vi "SFCS_ChkRout.vi"(5 "URL":string) -> (1 "Status":string)   [LabVIEW 2011]
uses:
  Instance           4 29Saved   SFCS_ChkRoute_ComCode .vi
  Instance           1 29Saved   SFCS_ChkRoute_ComCode .vi
  Instance           2 29Saved   SFCS_ChkRoute_ComCode .vi
  Instance           3 29Saved   SFCS_ChkRoute_ComCode .vi
  data/MCSDLL.dll
panel:
  out "軟體版本Software Version":string
  out "Begin time":u32
  out "SFCS System Enable":string
  out "STAGE":string
  out "Unit SN":string
  out "USN_Length":i32
  out "SFCS_IP":string
  # "SFCS Check Route"
  # "2015-3-27"
  # "SFCS的網址"
  # "站名"
  # "序號"
  # "訊息"
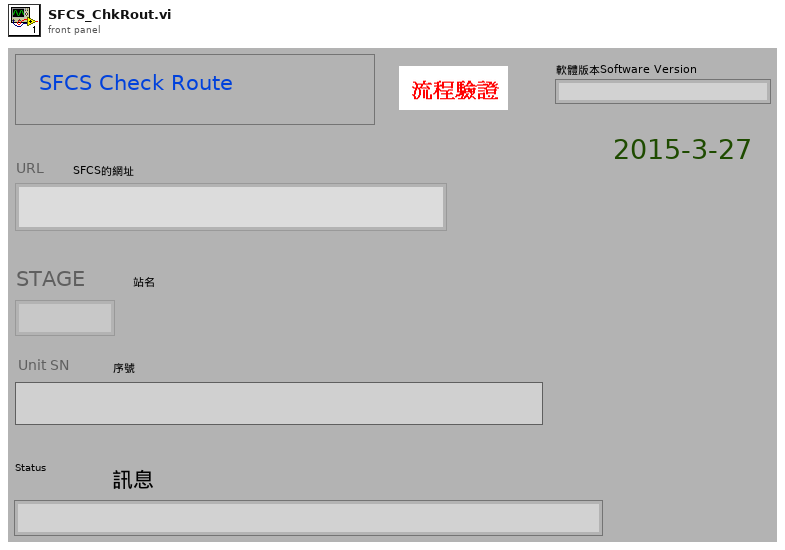
[diagram p1: front panel]
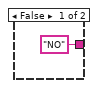
[diagram p5: hidden frame]
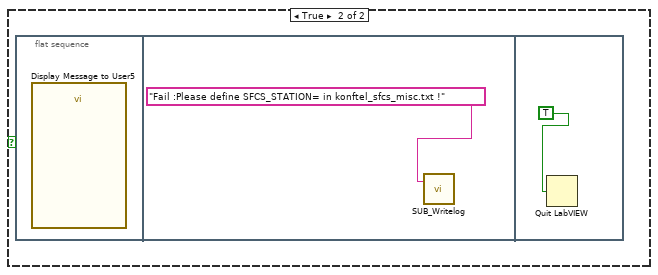
[diagram p8: hidden frame]
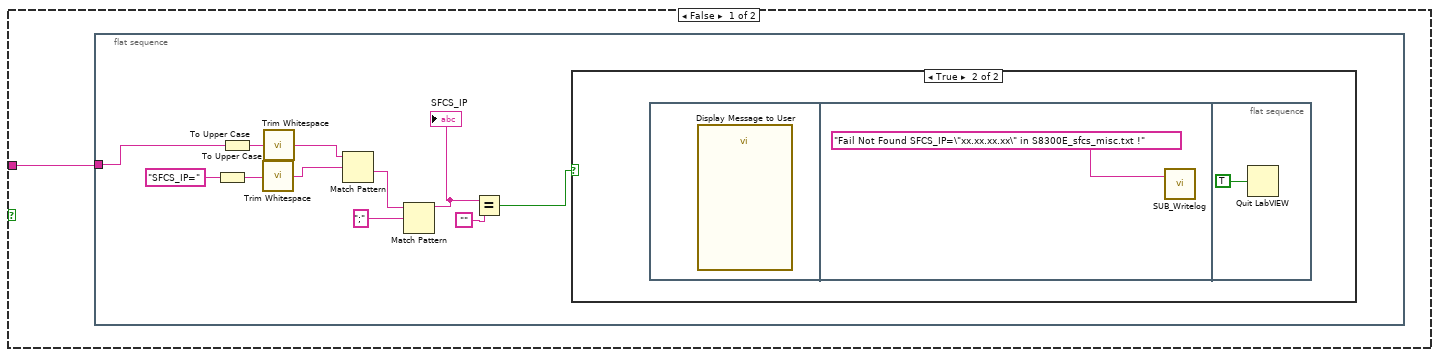
[diagram p10: hidden frame]
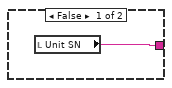
[diagram p12: hidden frame]
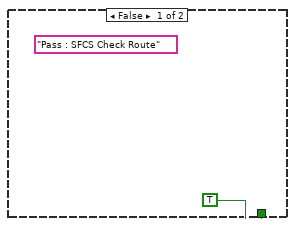
[diagram p13: hidden frame]
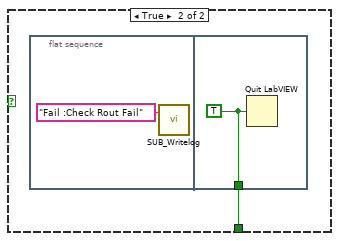
[diagram p14: hidden frame]
diagram:
  n1 = flat-sequence {
    frame #0 {
      n2 = Tick Count (ms)() -> (millisecond timer value=→"Begin time":u32)
    }
    frame #1 {
      n3 = call "SUB_SW_Version.vi"() -> ("Current Software Version"=→"軟體版本Software Version":string)  [unwired: 3 in]
      n4 = local write "Unit SN"("") -> ()
    }
    frame #2 {
      n5 = call "SUB_ReadScript_File.vi"("Script FileName"="barcode.log" ("name or relative path")) -> ("text"=w4:string, "error out"=w7:errorcluster)  [unwired: 1 in, 1 out]
      n6 = Unbundle(w7) -> ("code"=w6:i32)  [unwired: 2 out]
      n7 = Equal To 0?(x=w6) -> (x = 0?=w5:bool)
      n8 = case shown="True" w5 {
        tunnel: w4 -> [_ w11]
        frame False {
        }
        frame True {
          n9 = call "SUB_FindSpecificString.vi"("Find this String"="PRODUCT_SN=", "String data"=w11) -> ("before \"; \" string"=w9:string, "Found"=w10:bool)  [unwired: 2 in]
          n10 = case shown="True" w10 {
            tunnel: w9 -> [_ w13]
            frame False {
            }
            frame True {
              n11 = local write "Unit SN"(w13) -> ()
            }
          }
        }
      }
    }
    frame #3 {
      # "Check SFCS Enable in Mojo_script.txt"
      n12 = call "SUB_ReadScript_File.vi"("Script FileName"="S8300E_sfcs_misc.txt") -> ("text"=w19:string, "error out"=w16:errorcluster)  [unwired: 1 in, 1 out]
      n13 = Unbundle By Name(w16) -> ("code"=w17:i32)
      n14 = Equal To 0?(x=w17) -> (x = 0?=w18:bool)
      n15 = case shown="True" w18 {
        tunnel: w19 -> [_ w27]
        tunnel: ["NO" ("before \"; \" string") w25] -> w20
        frame False {
        }
        frame True {
          n16 = call "SUB_FindSpecificString.vi"("Find this String"="SFCS_SYSTEM_ENABLE=", "String data"=w27) -> ("before \"; \" string"=w25:string)  [unwired: 2 in, 1 out]
          "SFCS System Enable" <- w25
        }
      }
      n17 = Equal?(x=w20, y="YES") -> (x = y?=w15:bool)
      n18 = case shown="False" w15 {
        frame False {
          n19 = flat-sequence {
            frame #0 {
              n20 = call "SUB_Writelog.vi"("Pass/Fail"="Done :SFCS_ChkRoute_ComCode by PASS!") -> ()  [unwired: 2 in]
            }
            frame #1 {
              n21 = Quit LabVIEW(quit? (T)=TRUE) -> ()
            }
          }
        }
        frame True {
        }
      }
    }
    frame #4 {
      n22 = case shown="True" FALSE {
        frame False {
        }
        frame True {
          n23 = call "SUB_DELETE_SpecificFile.vi"("Filename to be  Deleted"="SFCS_INFO.LOG") -> ()  [unwired: 2 in, 1 out]
        }
      }
    }
    frame #5 {
      n24 = call "SUB_ReadScript_File.vi"("Script FileName"="S8300E_sfcs_misc.txt") -> ("text"=w31:string, "error out"=w34:errorcluster)  [unwired: 1 in, 1 out]
      n25 = Unbundle By Name(w34) -> ("code"=w33:i32)
      n26 = Equal To 0?(x=w33) -> (x = 0?=w32:bool)
      n27 = case shown="True" w32 {
        tunnel: w31 -> [_ w35]
        frame False {
        }
        frame True {
          n28 = To Upper Case(1:"SFCS_USNLength=" ("string")) -> (0:w44:string)
          n29 = To Upper Case(1:w35) -> (0:w46:string)
          n30 = call <vilib>:"Trim Whitespace.vi"("string"=w44) -> ("trimmed string"=w42:string)  [unwired: 1 in]
          n31 = call <vilib>:"Trim Whitespace.vi"("string"=w46) -> ("trimmed string"=w45:string)  [unwired: 1 in]
          n32 = Match Pattern(string=w45, regular expression=w42) -> (after substring=w40:string)  [unwired: 1 in, 3 out]
          n33 = Match Pattern(string=w40, regular expression=";") -> (before substring=w37:string)  [unwired: 1 in, 3 out]
          n34 = Equal?(x=w37, y="") -> (x = y?=w38:bool)
          n35 = Decimal String To Number(string=w37) -> (number=→"USN_Length":i32)  [unwired: 2 in, 1 out]
          n36 = case shown="False" w38 {
            tunnel: w35 -> [w50 _]
            frame False {
              n37 = To Upper Case(1:"SFCS_STATION=" ("string")) -> (0:w55:string)
              n38 = To Upper Case(1:w50) -> (0:w57:string)
              n39 = call <vilib>:"Trim Whitespace.vi"("string"=w55) -> ("trimmed string"=w53:string)  [unwired: 1 in]
              n40 = call <vilib>:"Trim Whitespace.vi"("string"=w57) -> ("trimmed string"=w56:string)  [unwired: 1 in]
              n41 = Match Pattern(string=w56, regular expression=w53) -> (after substring=w51:string)  [unwired: 1 in, 3 out]
              n42 = Match Pattern(string=w51, regular expression=";") -> (before substring=w49:string)  [unwired: 1 in, 3 out]
              "STAGE" <- w49
              n43 = Equal?(x=w49, y="") -> (x = y?=w47:bool)
              n44 = case shown="False" w47 {
                frame False {
                }
                frame True {
                  n45 = flat-sequence {
                    frame #0 {
                      n46 = call "Display Message to User5"() -> ()  [unwired: 10 in, 2 out]
                    }
                    frame #1 {
                      n47 = call "SUB_Writelog.vi"("Pass/Fail"="Fail :Please define SFCS_STATION= in konftel_sfcs_misc.txt !") -> ()  [unwired: 2 in]
                    }
                    frame #2 {
                      n48 = Quit LabVIEW(quit? (T)=TRUE) -> ()
                    }
                  }
                }
              }
            }
            frame True {
            }
          }
        }
      }
    }
    frame #6 {
      n49 = call "SUB_ReadScript_File.vi"("Script FileName"="S8300E_sfcs_misc.txt") -> ("text"=w61:string, "error out"=w64:errorcluster)  [unwired: 1 in, 1 out]
      n50 = Unbundle By Name(w64) -> ("code"=w63:i32)
      n51 = Not Equal To 0?(x=w63) -> (x != 0?=w62:bool)
      n52 = case shown="True" w62 {
        tunnel: w61 -> [w65 _]
        frame False {
          n53 = flat-sequence {
            tunnel: w65 -> [w71]
            frame #0 {
              n54 = To Upper Case(1:"SFCS_IP=" ("string")) -> (0:w75:string)
              n55 = To Upper Case(1:w71) -> (0:w76:string)
              n56 = call <vilib>:"Trim Whitespace.vi"("string"=w75) -> ("trimmed string"=w73:string)  [unwired: 1 in]
              n57 = call <vilib>:"Trim Whitespace.vi"("string"=w76) -> ("trimmed string"=w72:string)  [unwired: 1 in]
              n58 = Match Pattern(string=w72, regular expression=w73) -> (after substring=w70:string)  [unwired: 1 in, 3 out]
              n59 = Match Pattern(string=w70, regular expression=";") -> (before substring=w68:string)  [unwired: 1 in, 3 out]
              "SFCS_IP" <- w68
              n60 = Equal?(x=w68, y="") -> (x = y?=w66:bool)
              n61 = case shown="True" w66 {
                frame False {
                }
                frame True {
                  n62 = flat-sequence {
                    frame #0 {
                      n63 = call "Display Message to User"() -> ()  [unwired: 10 in, 2 out]
                    }
                    frame #1 {
                      n64 = call "SUB_Writelog.vi"("Pass/Fail"="Fail Not Found SFCS_IP=\"xx.xx.xx.xx\" in S8300E_sfcs_misc.txt !") -> ()  [unwired: 2 in]
                    }
                    frame #2 {
                      n65 = Quit LabVIEW(quit? (T)=TRUE) -> ()
                    }
                  }
                }
              }
            }
          }
        }
        frame True {
          n66 = flat-sequence {
            frame #0 {
              n67 = call "Display Message to User2"() -> ()  [unwired: 10 in, 2 out]
            }
            frame #1 {
              n68 = call "SUB_Writelog.vi"("Pass/Fail"="Fail S8300E_sfcs_misc.txt  Missing!") -> ()  [unwired: 2 in]
            }
            frame #2 {
              n69 = Quit LabVIEW(quit? (T)=TRUE) -> ()
            }
          }
        }
      }
    }
    frame #7 {
      n70 = local read "SFCS_IP"() -> (w81:string)
      n71 = local write "URL"(w81) -> ()
    }
    frame #8 {
      n72 = while {
        stop <- w83 stop-if-true
        n73 = flat-sequence {
          tunnel: [w87] -> w82
          tunnel: [w91] -> w83
          tunnel: w82 -> [w90]
          frame #0 {
            n74 = local read "Unit SN"() -> (w86:string)
            n75 = String Length(string=w86) -> (length=w85:i32)
            n76 = Equal To 0?(x=w85) -> (x = 0?=w84:bool)
            n77 = case shown="True" w84 {
              tunnel: [w88 w89] -> w87
              frame False {
                n78 = local read "Unit SN"() -> (w88:string)
              }
              frame True {
                n79 = call "Prompt User for Input"() -> ("Unit SN"=w89:string)  [unwired: 17 in, 2 out]
                "Unit SN" <- w89
              }
            }
          }
          frame #1 {
            n80 = local read "STAGE"() -> (w102:string)
            n81 = dll-call lib="D:/S8300E-Project/data/MCSDLL.dll" fn="SFCS_CheckRoute"("URL"="URL", "SN"=w90, "Stage"=w102) -> (w93:string)  [unwired: 6 in, 2 out]
            "Status" <- w93
            n82 = To Upper Case(1:"OK" ("string")) -> (0:w99:string)
            n83 = To Upper Case(1:w93) -> (0:w101:string)
            n84 = call <vilib>:"Trim Whitespace.vi"("string"=w99) -> ("trimmed string"=w96:string)  [unwired: 1 in]
            n85 = call <vilib>:"Trim Whitespace.vi"("string"=w101) -> ("trimmed string"=w100:string)  [unwired: 1 in]
            n86 = Match Pattern(string=w100, regular expression=w96) -> (match substring=w97:string)  [unwired: 1 in, 3 out]
            n87 = Not Equal?(x=w97, y=w96) -> (x != y?=w95:bool)
            n88 = Concatenate Strings("系統訊息" ("string"), w93) -> (w92:string)
            n89 = case shown="True" w95 {
              tunnel: w92 -> [_ w110]
              tunnel: [TRUE w109] -> w91
              frame False {
                (unwired) "Pass : SFCS Check Route" ("Pass/Fail")
              }
              frame True {
                n90 = call "SUB_YESNO.vi"("Debug View"=w110, "Status"="網路線有插好 ?") -> ("yes/no"=w107:enum32{"No Selection", "Yes", "No", "None"})  [unwired: 1 in]
                n91 = Equal?(x=w107, y=enum32{"No Selection", "Yes", "No", "None"}."No") -> (x = y?=w105:bool)
                n92 = case shown="False" w105 {
                  tunnel: [w111 w114] -> w109
                  frame False {
                    n93 = flat-sequence {
                      tunnel: [FALSE] -> w111
                      frame #0 {
                        n94 = local write "Unit SN"("") -> ()
                      }
                      frame #1 {
                      }
                    }
                  }
                  frame True {
                    n95 = flat-sequence {
                      tunnel: [w116] -> w114
                      frame #0 {
                        n96 = call "SUB_Writelog.vi"("Pass/Fail"="Fail :Check Rout Fail") -> ()  [unwired: 2 in]
                      }
                      frame #1 {
                        w116 = TRUE ("quit? (T)")
                        n97 = Quit LabVIEW(quit? (T)=w116) -> ()
                      }
                    }
                  }
                }
              }
            }
          }
        }
      }
    }
    frame #9 {
      n98 = flat-sequence {
        tunnel: [w118] -> w117
        tunnel: w117 -> [w126]
        frame #0 {
          n99 = local read "Unit SN"() -> (w120:string)
          n100 = Concatenate Strings("USN=" ("string"), w120, ";", "\r") -> (w118:string)
          n101 = call "SUB_WrteSFCS_INFO.vi"("Pass/Fail"=w118) -> ()  [unwired: 2 in]
        }
        frame #1 {
          w125 = "\r"
          n102 = local read "Begin time"() -> (w130:u32)
          n103 = Tick Count (ms)() -> (millisecond timer value=w129:u32)
          n104 = call "SUB_CAL_TESTTIME.vi"("Test Item name"="SFCS_ChkRoute_ComCode", "Stop tick time"=w129, "Start tick time"=w130) -> ("Test Time output"=w124:string)  [unwired: 2 in]
          n105 = Concatenate Strings("Pass :SFCS_ChkRoute_ComCode" ("Pass/Fail"), w125, w126, w125, w124) -> (w123:string)
          n106 = call "SUB_Writelog.vi"("Pass/Fail"=w123) -> ()  [unwired: 2 in]
        }
        frame #2 {
          n107 = Request Deallocation(TRUE ("flag")) -> ()
        }
        frame #3 {
          n108 = Quit LabVIEW(quit? (T)=TRUE) -> ()
        }
      }
    }
  }
